vi "F-Domain Img Filter App.vi"() -> ()   [LabVIEW 2014]
doc: "This example shows how to apply a lookup table to an image. Lookup table (LUT) transformations are basic mathematical functions that can be used to improve the contrast and brightness of an image by modifying the intensity dynamics of regions with poor contrast. The LUT can also be used to highlight details in areas containing significant information. In NI Vision, apart from the predefined functions that can be used through the IMAQ MathLookup VI, you can also apply your own lookup tables using the IMAQ UserLookup VI."
uses:
  <vilib>/vision/NI_Vision_Development_Module.lvlib
panel:
  in  "Size & Order #":T1={"X Size"=3, "Y Size"=3, "Order #"=4}
  in  "Size & Tolerance":T2={"X Size"=3, "Y Size"=3, "% Tolerance"=40}
  in  "Kernel#":i32
  in  "Order":i32=3
  in  "Filter":i32(listbox)
  in  "Stop Button":bool
  out "Dst":T3(plugin-control) caption="Lut Image"
  out "Image Source":T3(plugin-control)
  # "Configuration"
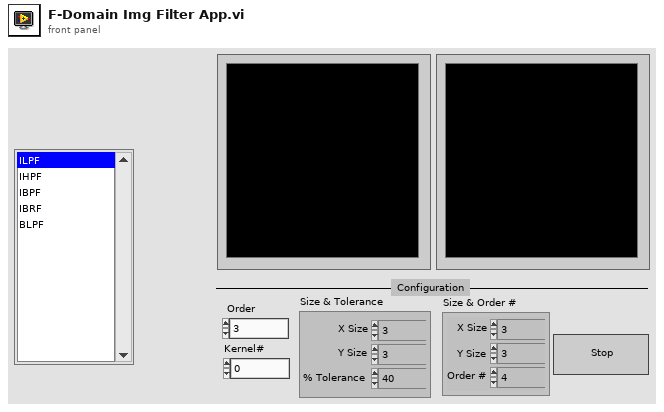
[diagram p1: front panel]
types:
  T1 = cluster{"X Size":i32, "Y Size":i32, "Order #":i32}
  T2 = cluster{"X Size":i32, "Y Size":i32, "% Tolerance":i32}
  T3 = typedef "IMAQ Image.ctl" = refnum<image>
  T4 = cluster{"Filter":string, "Kernel Size":i32, "Kernel Number":i32, "Size & Tolerance":cluster{"X Size":i32, "Y Size":i32, "% Tolerance":i32}, "Size & Order #":cluster{"X Size":i32, "Y Size":i32, "Order #":i32}}
  T5 = typedef "Image Type" = u32
  T6 = cluster{"Filter":i32, "Order":i32, "Kernel#":i32, "Size & Tolerance":cluster{"X Size":i32, "Y Size":i32, "% Tolerance":i32}, "Size & Order #":cluster{"X Size":i32, "Y Size":i32, "Order #":i32}}
  T7 = enum32{"Differentiation", "Gradient", "Prewitt", "Roberts", "Sigma", "Sobel"}
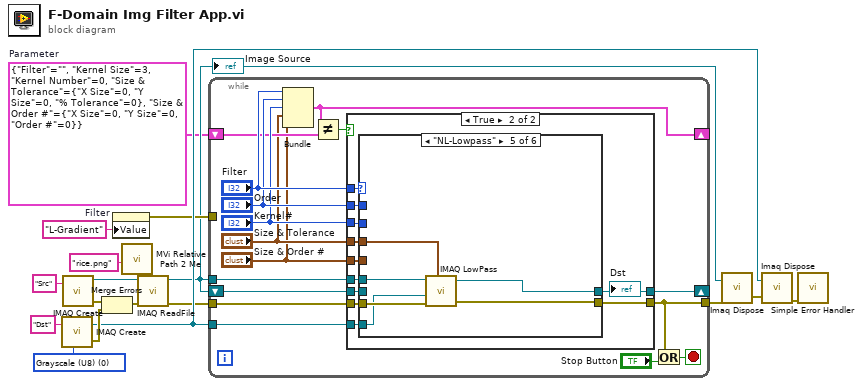
[diagram p0: block diagram]
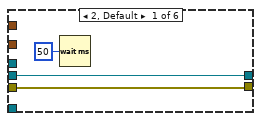
[diagram p3: hidden frame]
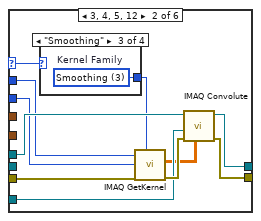
[diagram p4: hidden frame]
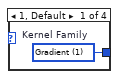
[diagram p5: hidden frame]
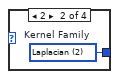
[diagram p6: hidden frame]
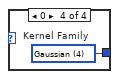
[diagram p7: hidden frame]
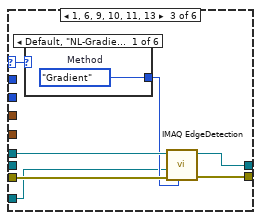
[diagram p8: hidden frame]
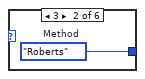
[diagram p9: hidden frame]
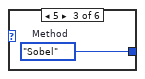
[diagram p10: hidden frame]
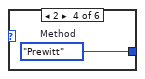
[diagram p11: hidden frame]
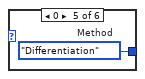
[diagram p12: hidden frame]
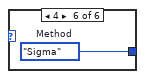
[diagram p13: hidden frame]
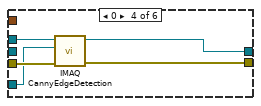
[diagram p14: hidden frame]
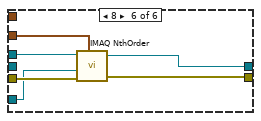
[diagram p15: hidden frame]
diagram:
  w2 = T4 {"Filter"="", "Kernel Size"=3, "Kernel Number"=0, "Size & Tolerance"={"X Size"=0, "Y Size"=0, "% Tolerance"=0}, "Size & Order #"={"X Size"=0, "Y Size"=0, "Order #"=0}}  # Parameter
  w14 = T5 0 items=["Grayscale (U8)", "Grayscale (I16)", "Grayscale (SGL)", "Complex (CSG)", "RGB (U32)", "HSL (U32)", "RGB (U64)", "Grayscale (U16)"] ("Image Type")
  n1 = call "IMAQ Create"("Image Name"="Dst", "Image Type"=w14) -> ("New Image"=w9:T3, "error out"=w13:errorcluster)  [unwired: 3 in]
  n2 = call "IMAQ Create"("Image Name"="Src") -> ("New Image"=w17:T3, "error out"=w11:errorcluster)  [unwired: 4 in]
  n3 = Merge Errors(w11, w13) -> (w12:errorcluster)
  n4 = property on="Filter" class="LstBox (strict)"("Value"="L-Gradient" ("Filter")) -> (error out=w4:errorcluster)  [unwired: 2 in, 1 out]
  n5 = call "MVi Relative Path 2 Me.vi"("Relative Path"="rice.png" ("name or relative path")) -> ("Appended Dir"=w6:path)  [unwired: 5 in, 1 out]
  n6 = call "IMAQ ReadFile"("File Path"=w6, "error in (no error)"=w12, "Image"=w17) -> ("error out"=w1:errorcluster, "Image Out"=w3:T3)  [unwired: 4 in, 3 out]
  "Image Source" <- w3
  n7 = while {
    tunnel: w1 -> [w34]
    tunnel: w3 -> [w33]
    tunnel: w9 -> [w32]
    tunnel: [w29] -> w10
    tunnel: w4 -> [_]
    shift-right: [w25] -> _
    shift-left: w2 -> [w24]
    shift-right: [w22] -> _
    shift-left: w3 -> [w21]
    stop <- w30 stop-if-true
    n8 = Bundle("Filter"="Filter", "Order"="Order", "Kernel#"="Kernel#", "Size & Tolerance"="Size & Tolerance", "Size & Order #"="Size & Order #") -> (w25:T6)  [unwired: 1 in]
    n9 = Not Equal?(x=w25, y=w24) -> (x != y?=w23:bool)
    n10 = case shown="True" w23 {
      tunnel: w34 -> [w36 w47]
      tunnel: w33 -> [_ w46]
      tunnel: w32 -> [_ w45]
      tunnel: "Filter" -> [_ w44]
      tunnel: [w36 w39] -> w29
      tunnel: "Order" -> [_ w43]
      tunnel: "Kernel#" -> [_ w42]
      tunnel: [w35 w41] -> w22
      tunnel: w21 -> [w35 w40]
      tunnel: "Size & Tolerance" -> [_ w38]
      tunnel: "Size & Order #" -> [_ w37]
      frame False {
      }
      frame True {
        n11 = case shown="\"NL-Lowpass\"" w44 {
          selector: w44 -> [_ w56 w68 _ _ _]
          tunnel: w47 -> [w50 w61 w70 w82 w88 w93]
          tunnel: w46 -> [_ w58 w69 w80 w87 w92]
          tunnel: w45 -> [_ w53 w66 w81 w86 w91]
          tunnel: [w50 w59 w72 w83 w89 w95] -> w39
          tunnel: [w48 w57 w71 w79 w85 w94] -> w41
          tunnel: w43 -> [_ w54 _ _ _ _]
          tunnel: w42 -> [_ w51 _ _ _ _]
          tunnel: w40 -> [w48 _ _ _ _ _]
          tunnel: w38 -> [_ _ _ _ w84 _]
          tunnel: w37 -> [_ _ _ _ _ w90]
          frame 2, Default {
            n12 = Wait (ms)(milliseconds to wait=u32 50) -> ()  [unwired: 1 out]
          }
          frame 3, 4, 5, 12 {
            n13 = case shown="\"Smoothing\"" w56 {
              tunnel: [w62 w63 w64 w65] -> w55
              frame 1, Default {
                w62 = u16 1 items=["Gradient"=1, "Laplacian"=2, "Smoothing"=3, "Gaussian"=4]  # Kernel Family
              }
              frame 2 {
                w63 = u16 2 items=["Gradient"=1, "Laplacian"=2, "Smoothing"=3, "Gaussian"=4]  # Kernel Family
              }
              frame 3 {
                w64 = u16 3 items=["Gradient"=1, "Laplacian"=2, "Smoothing"=3, "Gaussian"=4]  # Kernel Family
              }
              frame 0 {
                w65 = u16 4 items=["Gradient"=1, "Laplacian"=2, "Smoothing"=3, "Gaussian"=4]  # Kernel Family
              }
            }
            n14 = call "IMAQ GetKernel"("Kernel Family"=w55, "error in (no error)"=w61, "Kernel Number"=w51, "Kernel Size (3,5,...)"=w54) -> ("error out"=w60:errorcluster, "Kernel"=w52:sgl[][])  [unwired: 4 in, 2 out]
            n15 = call "IMAQ Convolute"("Kernel"=w52, "error in (no error)"=w60, "Image Dst"=w53, "Image Src"=w58) -> ("error out"=w59:errorcluster, "Image Dst Out"=w57:T3)  [unwired: 6 in]
          }
          frame 1, 6, 9, 10, 11, 13 {
            n16 = case shown="Default, \"NL-Gradient\"" w68 {
              tunnel: [w73 w74 w75 w76 w77 w78] -> w67
              frame 1, Default {
                w73 = T7."Gradient"  # Method
              }
              frame 3 {
                w74 = T7."Roberts"  # Method
              }
              frame 5 {
                w75 = T7."Sobel"  # Method
              }
              frame 2 {
                w76 = T7."Prewitt"  # Method
              }
              frame 0 {
                w77 = T7."Differentiation"  # Method
              }
              frame 4 {
                w78 = T7."Sigma"  # Method
              }
            }
            n17 = call "IMAQ EdgeDetection"("Method"=w67, "error in (no error)"=w70, "Image Dst"=w66, "Image Src"=w69) -> ("error out"=w72:errorcluster, "Image Dst Out"=w71:T3)  [unwired: 6 in]
          }
          frame 0 {
            n18 = call "IMAQ CannyEdgeDetection"("Image Src"=w80, "Image Dst"=w81, "error in (no error)"=w82) -> ("Image Dst Out"=w79:T3, "error out"=w83:errorcluster)  [unwired: 5 in]
          }
          frame 7 {
            n19 = call "IMAQ LowPass"("Image Src"=w87, "Size & Tolerance"=w84, "Image Dst"=w86, "error in (no error)"=w88) -> ("Image Dst Out"=w85:T3, "error out"=w89:errorcluster)  [unwired: 3 in]
          }
          frame 8 {
            n20 = call "IMAQ NthOrder"("Image Src"=w92, "Size & Order #"=w90, "Image Dst"=w91, "error in (no error)"=w93) -> ("Image Dst Out"=w94:T3, "error out"=w95:errorcluster)  [unwired: 3 in]
          }
        }
        "Dst" <- w41
      }
    }
    n21 = Or(x=w29, y="Stop Button") -> (x .or. y?=w30:bool)
  }
  n22 = call "Imaq Dispose"("Image"=w3, "error in (no error)"=w10) -> ("error out"=w8:errorcluster)  [unwired: 4 in]
  n23 = call "Imaq Dispose"("Image"=w9, "error in (no error)"=w8) -> ("error out"=w16:errorcluster)  [unwired: 4 in]
  n24 = call <vilib>:"Simple Error Handler.vi"("error in (no error)"=w16) -> ()  [unwired: 4 in, 5 out]
